vi "cursor test 2.vi"() -> ()   [LabVIEW 2019]
panel:
  in  "Delete Cursor":bool
  in  "Add Cursor":bool
  out "XY Graph":cluster{dbl[], dbl[]}(graph)
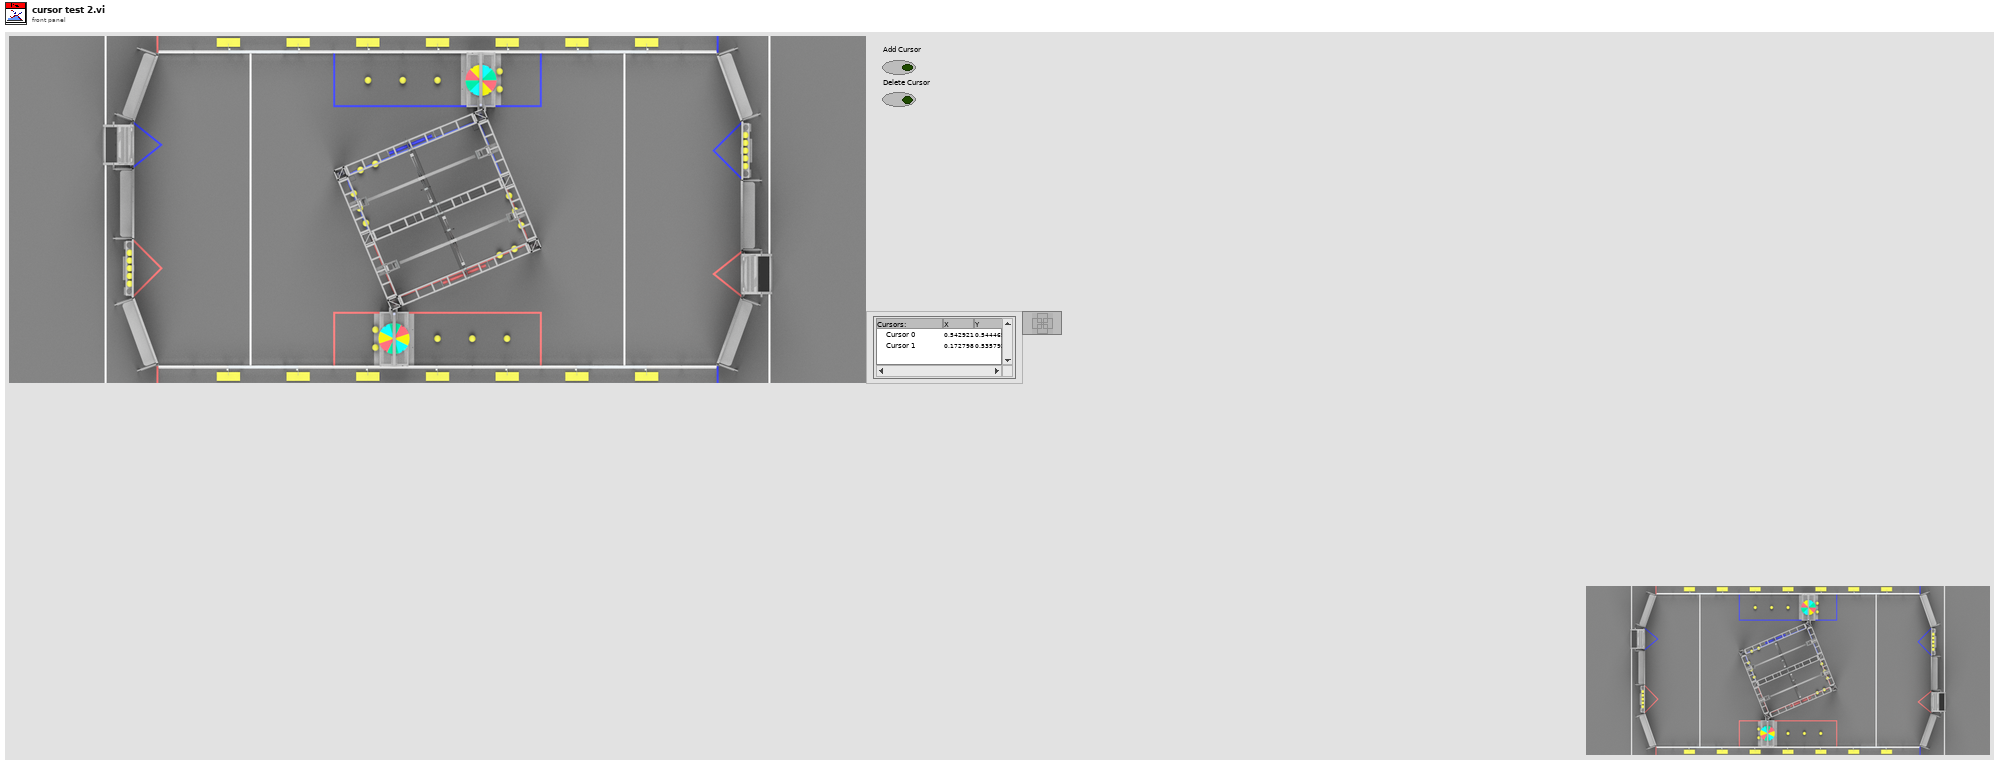
[diagram p1: front panel]
types:
  T1 = cluster{"Name":string, "Color":u32, "Style":u8, "Point Style":u8, "Name Visible":bool, "Allow Drag":bool, "Cursor Mode":u32, "Plot":i32, "Index":i32, "Position":cluster{"X":dbl, "Y":dbl}, "X Scale":u32, "Y Scale":u32, "Watch Plots":i32[], "Watch All Plots":bool, "Plot Area":i32, "Label Offset":cluster{"X":dbl, "Y":dbl}}
  T2 = typedef "LVCursorListTypeDef.ctl" = cluster{"Name":string, "Color":u32, "Style":u8, "Point Style":u8, "Name Visible":bool, "Allow Drag":bool, "Cursor Mode":u32, "Plot":i32, "Index":i32, "Position":cluster{"X":dbl, "Y":dbl}, "X Scale":u32, "Y Scale":u32, "Watch Plots":i32[], "Watch All Plots":bool, "Plot Area":i32, "Label Offset":cluster{"X":dbl, "Y":dbl}}[]
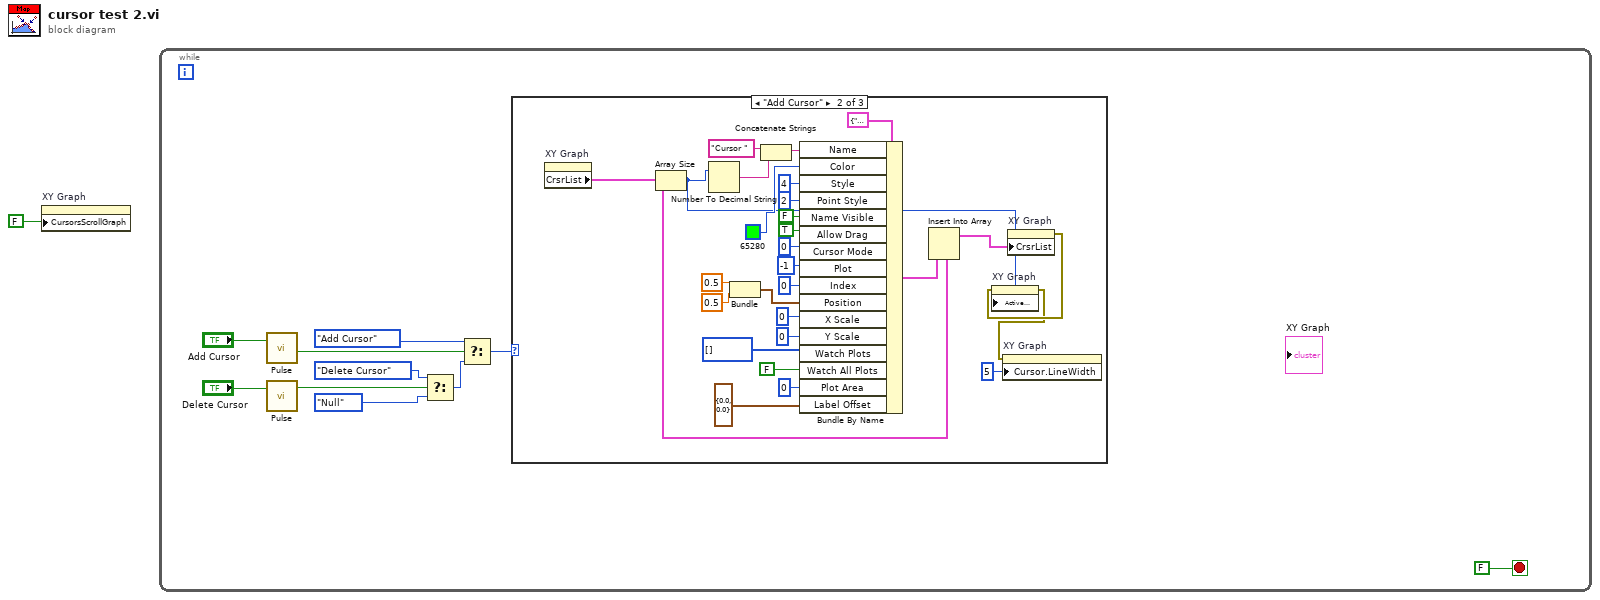
[diagram p0: block diagram]
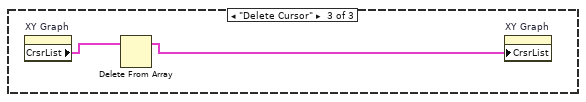
[diagram p3: hidden frame]
diagram:
  n1 = property on="XY Graph" class="XYGraph (strict)"("CursorsScrollGraph"=FALSE ("Cursors Scroll Graph")) -> ()  [unwired: 2 in, 2 out]
  n2 = while {
    stop <- FALSE stop-if-true
    n3 = call "Pulse.vi"("Input"="Add Cursor") -> ("Output"=w7:bool)  [unwired: 10 in]
    n4 = call "Pulse.vi"("Input"="Delete Cursor") -> ("Output"=w8:bool)  [unwired: 10 in]
    n5 = Select(t=enum16{"Null", "Add Cursor", "Delete Cursor"}."Delete Cursor", s=w8, f=enum16{"Null", "Add Cursor", "Delete Cursor"}."Null") -> (s? t:f=w4:enum16{"Null", "Add Cursor", "Delete Cursor"})
    n6 = Select(t=enum16{"Null", "Add Cursor", "Delete Cursor"}."Add Cursor", s=w7, f=w4) -> (s? t:f=w2:enum16{"Null", "Add Cursor", "Delete Cursor"})
    n7 = case shown="\"Add Cursor\"" w2 {
      frame "Null", Default {
      }
      frame "Add Cursor" {
        n8 = property on="XY Graph" class="XYGraph (strict)"() -> ("CrsrList"=w18:T2)  [unwired: 2 in, 2 out]
        n9 = Array Size(array=w18) -> (size(s)=w15:i32)
        n10 = Number To Decimal String(number=w15) -> (decimal integer string=w36:string)  [unwired: 1 in]
        n11 = Bundle(0.5, 0.5) -> (w21:cluster{dbl, dbl})  [unwired: 1 in]
        n12 = Concatenate Strings("Cursor ", w36) -> (w35:string)
        n13 = Bundle By Name(cluster=T1 {"Name"="", "Color"=33023, "Style"=0, "Point Style"=0, "Name Visible"=FALSE, "Allow Drag"=FALSE, "Cursor Mode"=0, "Plot"=0, "Index"=0, "Position"={"X"=0.0, "Y"=0.0}, "X Scale"=0, "Y Scale"=0, "Watch Plots"=[], "Watch All Plots"=FALSE, "Plot Area"=0, "Label Offset"={"X"=0.0, "Y"=0.0}} ("Cursor List"), "Name"=w35, "Color"=u32 65280, "Style"=u8 4, "Point Style"=u8 2, "Name Visible"=FALSE, "Allow Drag"=TRUE, "Cursor Mode"=u32 0, "Plot"=-1, "Index"=0, "Position"=w21, "X Scale"=u32 0, "Y Scale"=u32 0, "Watch Plots"=i32[] [], "Watch All Plots"=FALSE, "Plot Area"=0, "Label Offset"=cluster{"X":dbl, "Y":dbl} {"X"=0.0, "Y"=0.0}) -> (w39:T1)
        n14 = Insert Into Array(array=w18, new element=w39) -> (w38:T2)  [unwired: 1 in]
        n15 = property on="XY Graph" class="XYGraph (strict)"("CrsrList"=w38) -> (error out=w13:errorcluster)  [unwired: 2 in, 1 out]
        n16 = property on="XY Graph" class="XYGraph (strict)"(error in=w13, "Active Cursor"=w15) -> (error out=w12:errorcluster)  [unwired: 1 in, 1 out]
        n17 = property on="XY Graph" class="XYGraph (strict)"(error in=w12, "Cursor.LineWidth"=u8 5 ("Cursor.Line Width")) -> ()  [unwired: 1 in, 2 out]
      }
      frame "Delete Cursor" {
        n18 = property on="XY Graph" class="XYGraph (strict)"() -> ("CrsrList"=w41:T2)  [unwired: 2 in, 2 out]
        n19 = Delete From Array(array=w41) -> (array with subset deleted=w40:T2)  [unwired: 2 in, 1 out]
        n20 = property on="XY Graph" class="XYGraph (strict)"("CrsrList"=w40) -> ()  [unwired: 2 in, 2 out]
      }
    }
  }
